vi "Do Action.vi"(7 "Self Enqueuer":refnum<class "Message Enqueuer.lvclass">, 8 "error in (no error)":errorcluster, 11 "Change Failure Action in":refnum<class "Change Failure Action.lvclass">) -> (0 "error out":errorcluster)   [LabVIEW 2016, in "Assert API Components.lvlib" / "Assert Display.lvlib" / "Main Display.lvlib" / "Change Failure Action.lvclass"]
uses:
  Change Failure Action.lvclass
  <vilib>/ActorFramework/Message Enqueuer/Message Enqueuer.lvclass
  Assert API Components/Failure Actions.ctl
  Change Failure Action.lvclass/Change Failure Action.ctl
  Assert API Components/Assert API Components.lvlib
  Assert API Components/Log Assert Core Components/Log Assert Core.lvlib
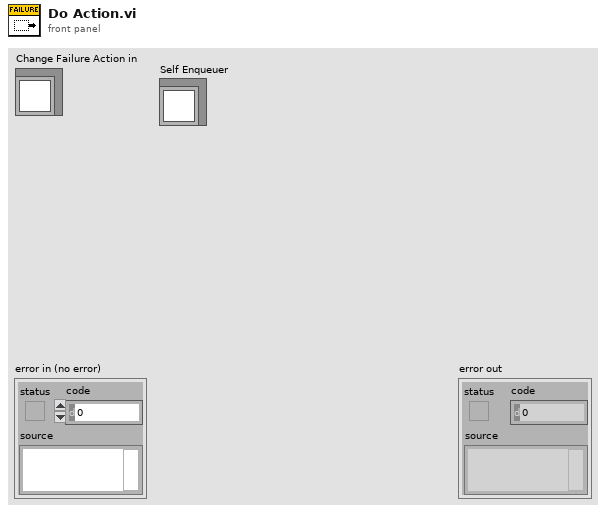
[diagram p1: front panel]
types:
  T1 = typedef "Assert API Components.lvlib/Failure Actions.ctl" = enum16{"None", "Log To File", "Pause Execution", "Abort Execution"}
  T2 = typedef "Assert API Components.lvlib/Log Assert Core.lvlib/Failure Action Change Event Reference.ctl" = cluster{"Failure Action Change Event":refnum<user-event>, "Event Registration Refnum":refnum<event-registration>}
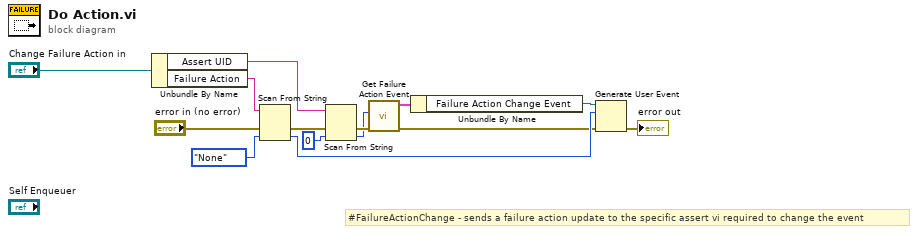
[diagram p0: block diagram]
diagram:
  # "#FailureActionChange - sends a failure action update to the specific assert vi required to change the event"
  n1 = Unbundle By Name("Change Failure Action in") -> ("Assert UID"=w8:string, "Failure Action"=w10:string)
  n2 = Scan From String(input string=w10, error in="error in (no error)", default 1=Failure_Actions."None" ("Default Failure Action")) -> (error out=w12:errorcluster, output 1=w3:T1)  [unwired: 2 in, 2 out]
  n3 = Scan From String(input string=w8, error in=w12, default 1=0) -> (error out=w7:errorcluster, output 1=w6:i32)  [unwired: 2 in, 2 out]
  n4 = call "Get Failure Action Event.vi"("error in (no error)"=w7, "Assert VI UID"=w6) -> ("error out"=w2:errorcluster, "Failure Action Event References"=w5:T2)  [unwired: 8 in]
  n5 = Unbundle By Name(w5) -> ("Failure Action Change Event"=w4:refnum<user-event>)
  n6 = Generate User Event(user event=w4, event data cluster=w3, error in=w2) -> (error out=→"error out":errorcluster)  [unwired: 1 in, 1 out]
